vi "KB-ljv7000data.vi"(11 "Measure Data 2":T1[](array[typedef]) {"Judge Result" items=["HI"=1, "GO"=2, "LO"=4, "ALARM"=5]; "Data Info" items=["VALID", "ALARM", "WAIT"]}) -> (1 "外圆到平面的高度差":string, 2 "內圆高度差":string, 3 "内外圆高度差":string)   [LabVIEW 2015]
uses:
  LJ-V7000/Public/Clusters/Measure Data.ctl
  LJ-V7000/Public/constant/Measure Data Info.ctl
  LJ-V7000/Public/constant/Judge Result.ctl
  LJ-V7000/Keyence LJ-V7000.lvlib
panel:
  out "外平面":T1={"Data Info"=0, "Judge Result"=1, "reserve"=0, "reserve"=0, "Value"=0.0} {"Judge Result" items=["HI"=1, "GO"=2, "LO"=4, "ALARM"=5]; "Data Info" items=["VALID", "ALARM", "WAIT"]}
  out "ƒÈÔ²2":T1={"Data Info"=0, "Judge Result"=1, "reserve"=0, "reserve"=0, "Value"=0.0} {"Judge Result" items=["HI"=1, "GO"=2, "LO"=4, "ALARM"=5]; "Data Info" items=["VALID", "ALARM", "WAIT"]}
  out "ƒÈÔ²1":T1={"Data Info"=0, "Judge Result"=1, "reserve"=0, "reserve"=0, "Value"=0.0} {"Judge Result" items=["HI"=1, "GO"=2, "LO"=4, "ALARM"=5]; "Data Info" items=["VALID", "ALARM", "WAIT"]}
  out "外圆1 2":T1={"Data Info"=0, "Judge Result"=1, "reserve"=0, "reserve"=0, "Value"=0.0} {"Judge Result" items=["HI"=1, "GO"=2, "LO"=4, "ALARM"=5]; "Data Info" items=["VALID", "ALARM", "WAIT"]}
  out "外圆1":T1={"Data Info"=0, "Judge Result"=1, "reserve"=0, "reserve"=0, "Value"=0.0} {"Judge Result" items=["HI"=1, "GO"=2, "LO"=4, "ALARM"=5]; "Data Info" items=["VALID", "ALARM", "WAIT"]}
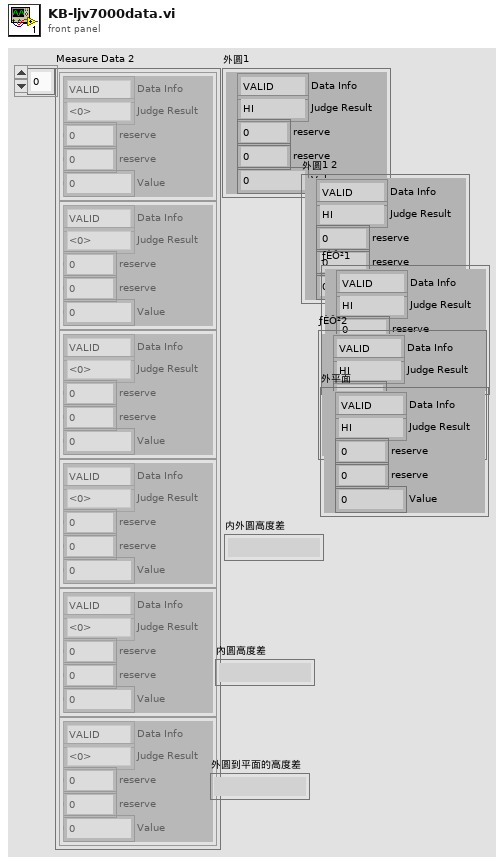
[diagram p1: front panel]
types:
  T1 = typedef "Keyence LJ-V7000.lvlib/Measure Data.ctl" = cluster{"Data Info":T2, "Judge Result":T3, "reserve":u8, "reserve":u8, "Value":sgl}
  T2 = typedef "Keyence LJ-V7000.lvlib/Measure Data Info.ctl" = u8
  T3 = typedef "Keyence LJ-V7000.lvlib/Judge Result.ctl" = u8
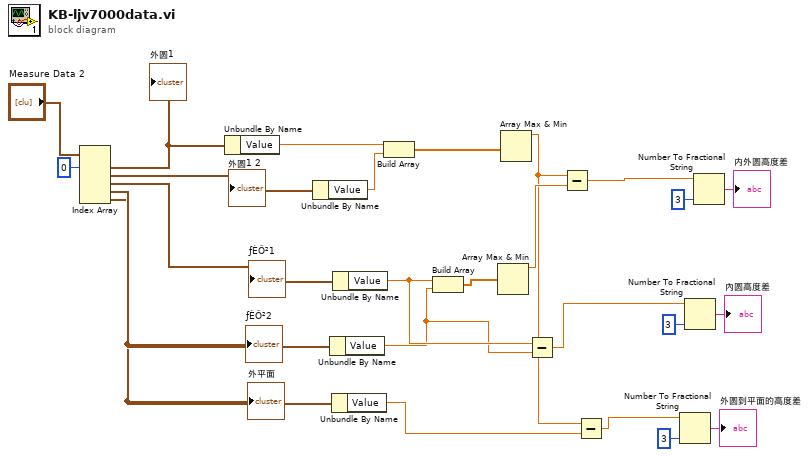
[diagram p0: block diagram]
diagram:
  n1 = Index Array(array="Measure Data 2", index #1=0 ("索引")) -> (element #1=w23:T1, element #2=w22:T1, element #3=w21:T1, element #4=w20:T1, element #5=w19:T1)  [unwired: 4 in]
  "外圆1" <- w23
  "外圆1 2" <- w22
  "ƒÈÔ²1" <- w21
  "ƒÈÔ²2" <- w20
  "外平面" <- w19
  n2 = Unbundle By Name(w23) -> ("Value"=w18:sgl)
  n3 = Unbundle By Name(w22) -> ("Value"=w17:sgl)
  n4 = Unbundle By Name(w20) -> ("Value"=w9:sgl)
  n5 = Unbundle By Name(w19) -> ("Value"=w2:sgl)
  n6 = Unbundle By Name(w21) -> ("Value"=w10:sgl)
  n7 = Build Array(w18, w17) -> (w16:sgl[])
  n8 = Build Array(w10, w9) -> (w15:sgl[])
  n9 = Array Max & Min(array=w15) -> (max value=w14:sgl)  [unwired: 3 out]
  n10 = Array Max & Min(array=w16) -> (max value=w3:sgl)  [unwired: 3 out]
  n11 = Subtract(x=w10, y=w9) -> (x-y=w6:sgl)
  n12 = Subtract(x=w3, y=w14) -> (x-y=w13:sgl)
  n13 = Subtract(x=w3, y=w2) -> (x-y=w1:sgl)
  n14 = Number To Fractional String(number=w1, precision (6)=i16 3 ("精度(6)")) -> (F-format string=→"外圆到平面的高度差":string)  [unwired: 2 in]
  n15 = Number To Fractional String(number=w6, precision (6)=i16 3 ("精度(6)")) -> (F-format string=→"內圆高度差":string)  [unwired: 2 in]
  n16 = Number To Fractional String(number=w13, precision (6)=i16 3 ("精度(6)")) -> (F-format string=→"内外圆高度差":string)  [unwired: 2 in]
